vi "Plot_Select_Main_Plot.vi"(0 "Mode":enum16{"Initialize", "Run"}(ring), 1 "State in":i32, 2 "Spec plot":enum16{"Counts", "Ext", "Conc", "Auto"}(ring), 7 "Spectra":refnum<vi>, 9 "Counts":cluster{"Wavelength":dbl[], "Spectra":dbl[]}, 11 "Exts":cluster{"Wavelength":dbl[], "Extinction ":dbl[]}, 12 "First?":bool) -> (6 "Plots":cluster{"Wavelength":dbl[], "Extinction ":dbl[]})   [LabVIEW 2025]
uses:
  <vilib>/Utility/miscctls.llb/LVFormatAndPrecisionTypeDef.ctl
panel:
  in  "Ext Min/Max":cluster{"Ext Ch1 Min":dbl, "Ext Ch1 Max":dbl}={"Ext Ch1 Min"=0.0, "Ext Ch1 Max"=1e-07}
  in  "Counts Min/Max":T1={"Counts Ch1 Min"=0.0, "Counts Ch1 Max"=200000.0}
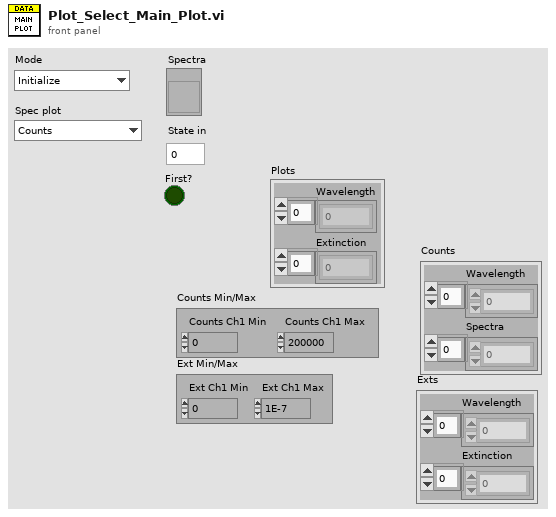
[diagram p1: front panel]
types:
  T1 = cluster{"Counts Ch1 Min":dbl, "Counts Ch1 Max":dbl}
  T2 = typedef "LVFormatAndPrecisionTypeDef.ctl" = cluster{"Format":u8, "Precision":u8}
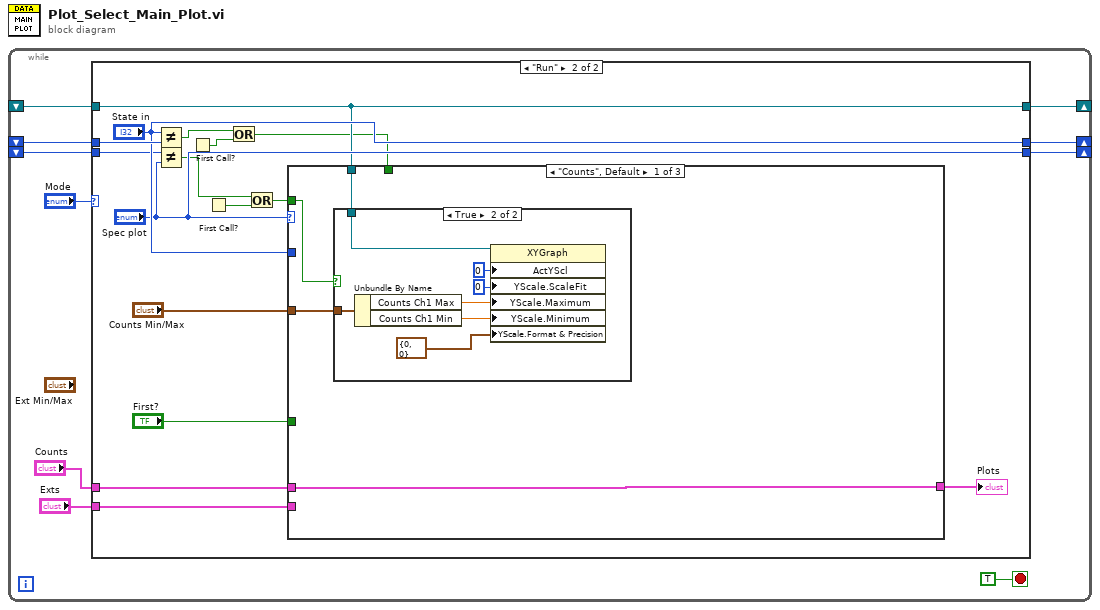
[diagram p0: block diagram]
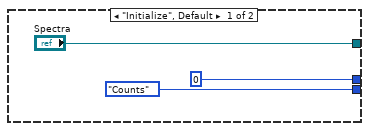
[diagram p2: hidden frame]
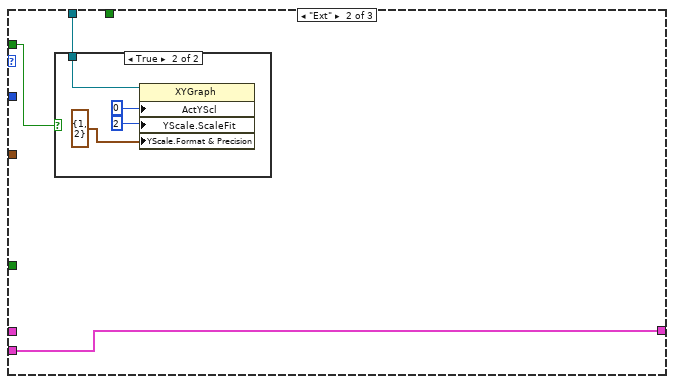
[diagram p4: hidden frame]
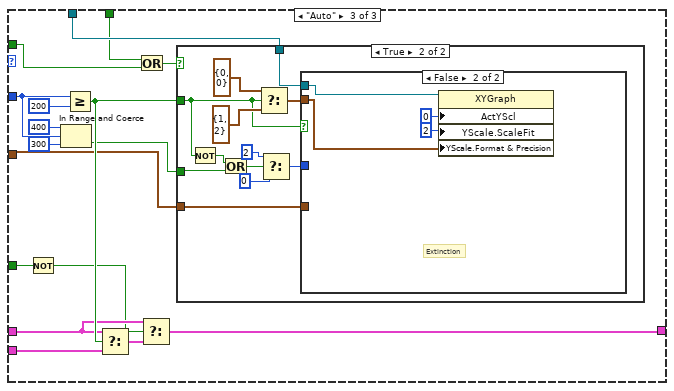
[diagram p6: hidden frame]
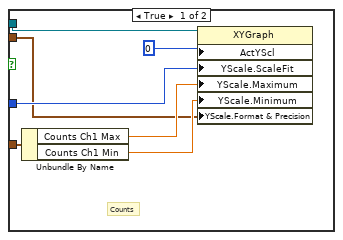
[diagram p8: hidden frame]
diagram:
  n1 = while {
    shift-right: [w8] -> _
    shift-left: _ -> [w7]
    shift-right: [w6] -> _
    shift-left: _ -> [w5]
    shift-right: [w4] -> _
    shift-left: _ -> [w3]
    stop <- TRUE stop-if-true
    n2 = case shown="\"Run\"" "Mode" {
      tunnel: [0 "State in"] -> w8
      tunnel: w7 -> [_ w29]
      tunnel: "Counts" -> [_ w28]
      tunnel: "Exts" -> [_ w27]
      tunnel: ["Spectra" w23] -> w6
      tunnel: w5 -> [_ w23]
      tunnel: [enum16{"Counts", "Ext", "Conc", "Auto"}."Counts" ("Spec plot") "Spec plot"] -> w4
      tunnel: w3 -> [_ w25]
      frame "Initialize", Default {
      }
      frame "Run" {
        n3 = Not Equal?(x="State in", y=w29) -> (x != y?=w19:bool)
        n4 = Not Equal?(x=w25, y="Spec plot") -> (x != y?=w17:bool)
        n5 = First Call?() -> (First Call?: T/F=w20:bool)
        n6 = First Call?() -> (First Call?: T/F=w16:bool)
        n7 = Or(x=w19, y=w20) -> (x .or. y?=w18:bool)
        n8 = Or(x=w17, y=w16) -> (x .or. y?=w15:bool)
        n9 = case shown="\"Counts\", Default" "Spec plot" {
          tunnel: w28 -> [w33 _ w53]
          tunnel: [w33 w43 w52] -> w14
          tunnel: w27 -> [_ w43 w63]
          tunnel: "State in" -> [_ _ w61]
          tunnel: w15 -> [w32 w41 w49]
          tunnel: w23 -> [w31 w42 w57]
          tunnel: "Counts Min/Max" -> [w30 _ w56]
          tunnel: w18 -> [_ _ w50]
          tunnel: "First?" -> [_ _ w55]
          frame "Counts", Default {
            n10 = case shown="True" w32 {
              tunnel: w31 -> [_ w40]
              tunnel: w30 -> [_ w38]
              frame False {
              }
              frame True {
                n11 = Unbundle By Name(w38) -> ("Counts Ch1 Max"=w37:dbl, "Counts Ch1 Min"=w36:dbl)
                n12 = property class="XYGraph"(reference=w40, "ActYScl"=0 ("Active Y Scale"), "YScale.ScaleFit"=u8 0 ("Y Scale.Scale Fit"), "YScale.Maximum"=w37, "YScale.Minimum"=w36, "YScale.Format & Precision"=T2 {"Format"=0, "Precision"=0} ("Y Scale.Display Format")) -> ()  [unwired: 1 in, 2 out]
              }
            }
          }
          frame "Ext" {
            n13 = case shown="True" w41 {
              tunnel: w42 -> [_ w47]
              frame False {
              }
              frame True {
                n14 = property class="XYGraph"(reference=w47, "ActYScl"=0 ("Active Y Scale"), "YScale.ScaleFit"=u8 2 ("Y Scale.Scale Fit"), "YScale.Format & Precision"=T2 {"Format"=1, "Precision"=2} ("Y Scale.Display Format")) -> ()  [unwired: 1 in, 2 out]
              }
            }
          }
          frame "Auto" {
            n15 = Not(x=w55) -> (.not. x?=w51:bool)
            n16 = In Range and Coerce(upper limit=400, x=w61, lower limit=300) -> (In Range?=w58:bool)  [unwired: 1 out]
            n17 = Greater Or Equal?(x=w61, y=200) -> (x >= y?=w62:bool)
            n18 = Select(t=w53, s=w62, f=w63) -> (s? t:f=w54:cluster{"Wavelength":dbl[], "Extinction ":dbl[]})
            n19 = Or(x=w50, y=w49) -> (x .or. y?=w48:bool)
            n20 = Select(t=w53, s=w51, f=w54) -> (s? t:f=w52:cluster{"Wavelength":dbl[], "Extinction ":dbl[]})
            n21 = case shown="True" w48 {
              tunnel: w62 -> [_ w69]
              tunnel: w58 -> [_ w76]
              tunnel: w57 -> [_ w68]
              tunnel: w56 -> [_ w66]
              frame False {
              }
              frame True {
                n22 = Not(x=w69) -> (.not. x?=w75:bool)
                n23 = Or(x=w75, y=w76) -> (x .or. y?=w74:bool)
                n24 = Select(t=T2 {"Format"=0, "Precision"=0} ("Y Scale.Display Format"), s=w69, f=T2 {"Format"=1, "Precision"=2} ("Y Scale.Display Format")) -> (s? t:f=w65:T2)
                n25 = Select(t=u8 2 ("Y Scale.Scale Fit"), s=w74, f=u8 0) -> (s? t:f=w67:u8)
                n26 = case shown="False" w69 {
                  tunnel: w68 -> [w80 w87]
                  tunnel: w67 -> [w79 _]
                  tunnel: w66 -> [w78 _]
                  tunnel: w65 -> [w77 w84]
                  frame True {
                    # "Counts"
                    n27 = Unbundle By Name(w78) -> ("Counts Ch1 Max"=w82:dbl, "Counts Ch1 Min"=w81:dbl)
                    n28 = property class="XYGraph"(reference=w80, "ActYScl"=0 ("Active Y Scale"), "YScale.ScaleFit"=w79, "YScale.Maximum"=w82, "YScale.Minimum"=w81, "YScale.Format & Precision"=w77) -> ()  [unwired: 1 in, 2 out]
                  }
                  frame False {
                    # "Extinction"
                    n29 = property class="XYGraph"(reference=w87, "ActYScl"=0 ("Active Y Scale"), "YScale.ScaleFit"=u8 2 ("Y Scale.Scale Fit"), "YScale.Format & Precision"=w84) -> ()  [unwired: 1 in, 2 out]
                  }
                }
              }
            }
          }
        }
        "Plots" <- w14
      }
    }
  }
